vi "Get Thread Configuration.vi"(8 "error in (no error)":errorcluster, 11 "Component Configuration in":refnum<class "Component Configurations.lvclass">) -> (0 "error out":errorcluster, 2 "Thread Configuration":refnum<class "Configuration.lvclass">, 3 "Component Configuration out":refnum<class "Component Configurations.lvclass">)   [LabVIEW 2019, in "DSF Core.lvlib" / "Component Configurations.lvclass"]
uses:
  Component Configurations.lvclass
  Configuration/Configuration.lvclass
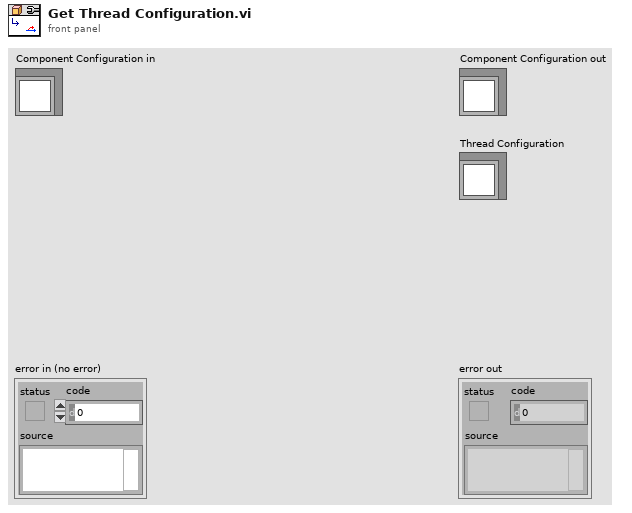
[diagram p1: front panel]
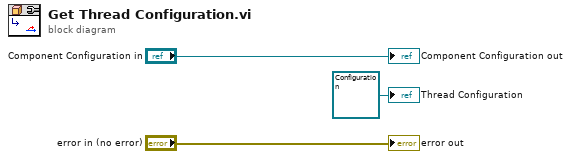
[diagram p0: block diagram]
diagram:
  "error out" <- "error in (no error)"
  "Component Configuration out" <- "Component Configuration in"
  "Thread Configuration" <- refnum<class "Configuration.lvclass"> refnum ("Thread Configuration")
